vi "RMS error check.vi"(8 "Threshold":dbl format="%#_13g", 9 "Z Axis":dbl[](array[numeric]), 10 "Y Axis":dbl[](array[numeric]), 11 "X Axis":dbl[](array[numeric])) -> (2 "Error?":bool[](array[boolean]), 3 "RMS":dbl[](array[numeric]))   [LabVIEW 2015]
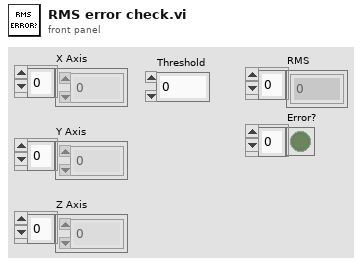
[diagram p1: front panel]
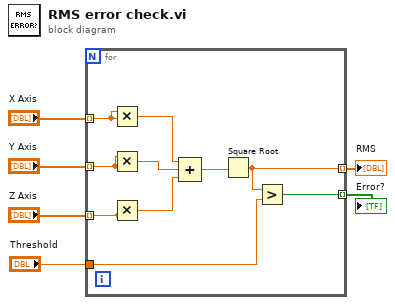
[diagram p0: block diagram]
diagram:
  n1 = for {
    tunnel: "X Axis" -> [w16] mode=indexing
    tunnel: "Y Axis" -> [w15] mode=indexing
    tunnel: "Z Axis" -> [w14] mode=indexing
    tunnel: "Threshold" -> [w9]
    tunnel: [w8] -> w1 mode=indexing
    tunnel: [w7] -> w2 mode=indexing
    n2 = Multiply(x=w16, y=w16) -> (x*y=w13:dbl)
    n3 = Multiply(x=w15, y=w15) -> (x*y=w12:dbl)
    n4 = Multiply(x=w14, y=w14) -> (x*y=w11:dbl)
    n5 = Compound Arithmetic op=ADD(w13, w12, w11) -> (w10:dbl)
    n6 = Square Root(x=w10) -> (sqrt(x)=w7:dbl)
    n7 = Greater?(x=w7, y=w9) -> (0:w8:bool)
  }
  "RMS" <- w2
  "Error?" <- w1
